vi "Initialize.vi"(7 "Custom Device Name":string, 8 "error in":errorcluster, 9 "Compiled Settings":variant, 10 "Custom Device API in":refnum<class "Custom Device API.lvclass">, 11 "Custom Device in":refnum<class "Template.lvclass">) -> (0 "error out":errorcluster, 3 "Custom Device out":refnum<class "Template.lvclass">)   [LabVIEW 2026, in "Template.lvlib" / "Template.lvclass"]
uses:
  Template.lvclass
  <userlib>/Custom Device Interfaces_v1.lvlibp/CustomDeviceAPI/Custom Device API.lvclass
  Types/TargetSettings.ctl
  Template.lvclass/Template.ctl
  Utilities/Get Output Channel Group.vi
  Utilities/Get Input Channel Group.vi
  Logging/Utilities/Log.Error.vi
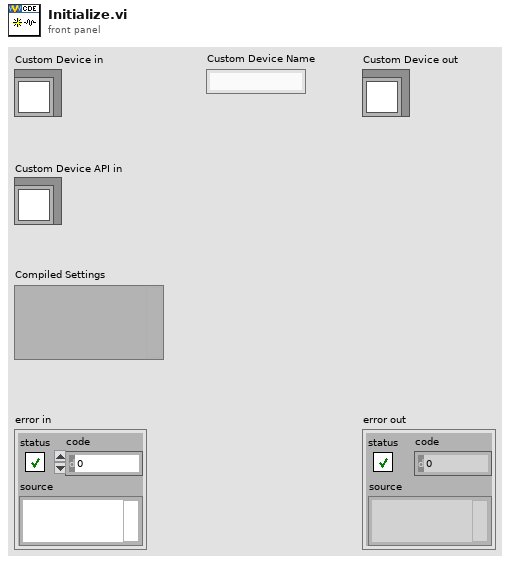
[diagram p1: front panel]
types:
  T1 = typedef "Template.lvlib/Template.lvclass/TargetSettings.ctl" = cluster{"Name":string}
  T2 = cluster{"Read":cluster{"Refs":cluster{"Data Reference":i32, "Offset":u64, "Length":u64}[], "Values":dbl[]}[], "Write":cluster{"Refs":cluster{"Data Reference":i32, "Offset":u64, "Length":u64}[], "Values":dbl[]}[], "ReadWrite":cluster{"Refs":i32[], "Values":dbl[], "Reset Values":dbl[]}[], "LUT":variant}
  T3 = cluster{"Refs":cluster{"Data Reference":i32, "Offset":u64, "Length":u64}[], "Values":dbl[]}
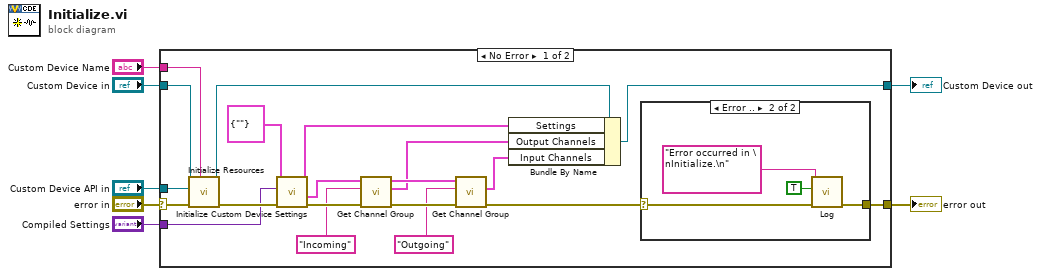
[diagram p0: block diagram]
diagram:
  n1 = case shown="No Error" "error in" {
    selector: "error in" -> [w27 w34]
    tunnel: "Custom Device in" -> [w19 w33]
    tunnel: "Custom Device API in" -> [w18 _]
    tunnel: [w17 w33] -> w3
    tunnel: [w22 w34] -> w6
    tunnel: "Compiled Settings" -> [w16 _]
    tunnel: "Custom Device Name" -> [w21 _]
    frame No Error {
      n2 = call "Initialize Resources.vi"("Custom Device Name"=w21, "error in"=w27, "Custom Device API in"=w18, "Custom Device in"=w19) -> ("error out"=w26:errorcluster, "Custom Device out"=w20:refnum<class "Template.lvclass">)  [unwired: 6 in]
      n3 = call "Initialize Custom Device Settings.vi"("error in"=w26, "Compiled Settings"=w16, "Custom Device Engine Settings in"=T1 {"Name"=""} ("Settings")) -> ("error out"=w25:errorcluster, "Channel Refs"=w13:T2, "Custom Device Engine Settings out"=w14:T1)  [unwired: 6 in]
      n4 = call-poly "Get Channel Group.vi"("error in"=w25, "Group Name"="Incoming", "Channel Refs"=w13) -> ("error out"=w24:errorcluster, "Channel Group"=w9:T3, "Channel Refs"=w11:T2)  [unwired: 6 in]
      n5 = call-poly "Get Channel Group.vi"("error in"=w24, "Group Name"="Outgoing", "Channel Refs"=w11) -> ("error out"=w23:errorcluster, "Channel Group"=w8:T3)  [unwired: 6 in, 1 out]
      n6 = Bundle By Name(cluster=w20, "Settings"=w14, "Output Channels"=w9, "Input Channels"=w8) -> (w17:refnum<class "Template.lvclass">)
      n7 = case shown="Error .." w23 {
        selector: w23 -> [w28 w31]
        tunnel: [w28 w30] -> w22
        frame No Error {
        }
        frame Error {
          n8 = call-poly "Log.vi"("error in"=w31, "Add to log file? (F)"=TRUE, "Message"="Error occurred in \nInitialize.\n" ("string")) -> ("error out"=w30:errorcluster)  [unwired: 8 in]
        }
      }
    }
    frame Error {
    }
  }
  "error out" <- w6
  "Custom Device out" <- w3
